vi "Read Elevation.vi"(8 "error in (no error)":errorcluster, 11 "AzElParameters in":refnum<class "AzElParameters.lvclass">) -> (0 "error out":errorcluster, 2 "Elevation.lvclass":refnum<class "Elevation.lvclass">, 3 "AzElParameters out":refnum<class "AzElParameters.lvclass">)   [LabVIEW 2022 SP3, in "TCSDataDefinitions.lvlib" / "TCSCommand.lvlib" / "TargetConfiguration.lvlib" / "Target.lvlib" / "FixedTarget.lvlib" / "AzElParameters.lvclass"]
uses:
  AzElParameters.lvclass
  Elevation/Elevation.lvclass
  AzElParameters.lvclass/AzElParameters.ctl
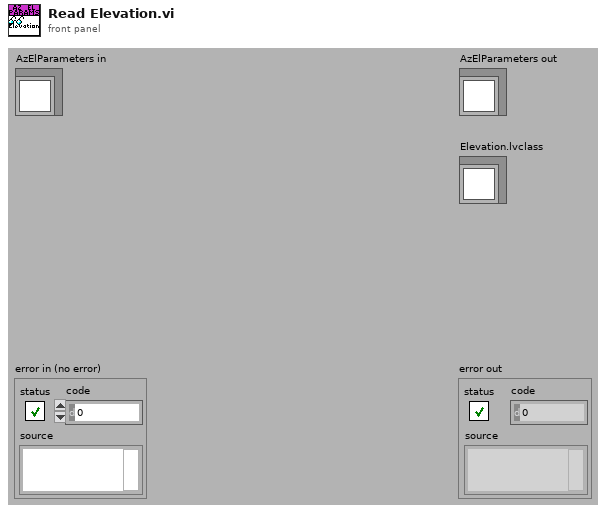
[diagram p1: front panel]
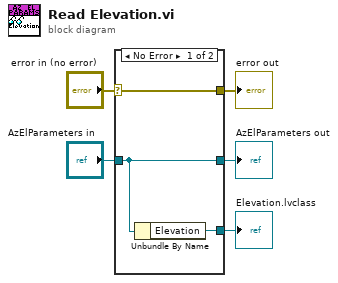
[diagram p0: block diagram]
diagram:
  n1 = case shown="No Error" "error in (no error)" {
    selector: "error in (no error)" -> [w8 w9]
    tunnel: [w8 w9] -> w4
    tunnel: [w7 w10] -> w2
    tunnel: "AzElParameters in" -> [w7 w10]
    tunnel: [w6 _] -> w1
    frame No Error {
      n2 = Unbundle By Name(w7) -> ("Elevation"=w6:refnum<class "Elevation.lvclass">)
    }
    frame Error {
    }
  }
  "error out" <- w4
  "AzElParameters out" <- w2
  "Elevation.lvclass" <- w1
